vi "DPS_Statemachine.vi"() -> ()   [LabVIEW 2015]
uses:
  <vilib>/express/express arith-compare/Formula/XNode/ExpressFormulaBlockNode.xnode
  State_DPS.ctl
  <vilib>/myRIO/Express VI/Onboard IO/I2C/I2C Express VI.xnode
  <vilib>/myRIO/Instrument Drivers/Onboard IO/I2C/vis/Configure.vi
  <vilib>/myRIO/Instrument Drivers/Onboard IO/I2C/I2C.lvlib
  <vilib>/myRIO/Instrument Drivers/Onboard IO/I2C/vis/Write.vi
  <vilib>/myRIO/Instrument Drivers/Onboard IO/I2C/typedefs/I2C Transfer Rate.ctl
  <vilib>/myRIO/Instrument Drivers/Onboard IO/I2C/typedefs/I2C User Configuration.ctl
  <vilib>/myRIO/Instrument Drivers/Onboard IO/I2C/typedefs/I2C Configuration.ctl
  <vilib>/myRIO/Common/Instrument Driver Framework/myRIO v1.0/I2C/typedefs/I2C Channels Enum.ctl
  <vilib>/myRIO/Common/Instrument Driver Framework/Utilities/typedefs/Generic FPGA Reference.ctl
  <vilib>/myRIO/Common/Instrument Driver Framework/Utilities/typedefs/myRIO v1.0 Reference.ctl
  <vilib>/myRIO/Common/Instrument Driver Framework/Utilities/typedefs/Hardware Version Enum.ctl
  <vilib>/myRIO/Common/Instrument Driver Framework/Utilities/typedefs/myRIO Generic Hardware Reference.ctl
  <vilib>/myRIO/Instrument Drivers/Onboard IO/I2C/typedefs/I2C Reference.ctl
  <vilib>/myRIO/Instrument Drivers/Onboard IO/I2C/vis/myRIO I2C Open.xnode
  <vilib>/myRIO/Common/Instrument Driver Framework/Utilities/vis/Is FPGA Ref Available.vi
  <vilib>/myRIO/Common/Instrument Driver Framework/myRIO v1.0/I2C/vis/myRIO v1.1 Open I2C.vi
  <vilib>/userdefined/High Color/nirio_resource_hc.ctl
panel:
  out "I2C error":errorcluster
  out "True Pressure":dbl
  in  "stop":bool
  out "True Temperature":dbl
  out "Uncompensated P":dbl
  in  "XLSB Read":dbl
  in  "OSS":dbl
  in  "MSB Read":dbl format="%#_13g"
  in  "LSB Read":dbl
  out "Uncompensated T":dbl format="%#_13g"
  out "error out":errorcluster
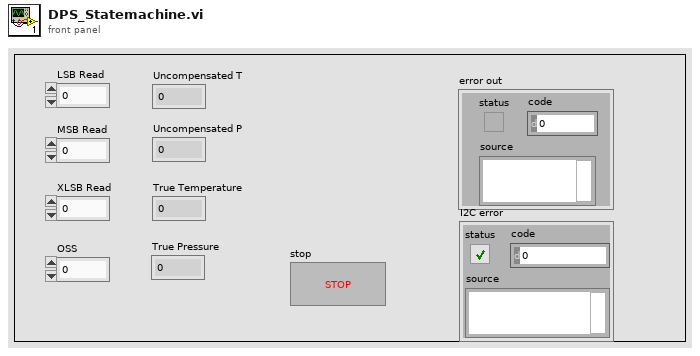
[diagram p1: front panel]
types:
  T1 = typedef "State_DPS.ctl" = enum16{"Read UT", "Wait", "Read & Calc UT", "Read UP", "Read & Calc UP", "Calculate TT", "Calculate TP"}
  T2 = typedef "I2C.lvlib/I2C Reference.ctl" = cluster{"myRIO Reference":T3, "I2C Channels Enum":T7, "I2C Configuration":T8}
  T3 = typedef "myRIO Generic Hardware Reference.ctl" = cluster{"myRIO Model":T4, "myRIO Hardware Reference":T5}
  T4 = typedef "Hardware Version Enum.ctl" = enum16{"Unknown", "myRIO-1900", "myRIO-1950", "roboRIO"}
  T5 = typedef "myRIO v1.0 Reference.ctl" = cluster{"Generic FPGA Reference":T6, "Allow multiple opens":bool}
  T6 = typedef "Generic FPGA Reference.ctl" = refnum<k20>
  T7 = typedef "I2C Channels Enum.ctl" = enum16{"Not Connected", "A/I2C", "B/I2C", "I2C/I2C"}
  T8 = typedef "I2C.lvlib/I2C Configuration.ctl" = cluster{"I2C Transfer Rate":T9}
  T9 = typedef "I2C.lvlib/I2C Transfer Rate.ctl" = enum16{"Standard mode (100 kbps)", "Fast mode (400 kbps)"}
  T10 = typedef "I2C.lvlib/I2C User Configuration.ctl" = cluster{"I2C Transfer Rate":T9}
  T11 = typedef "nirio_resource_hc.ctl" = tag
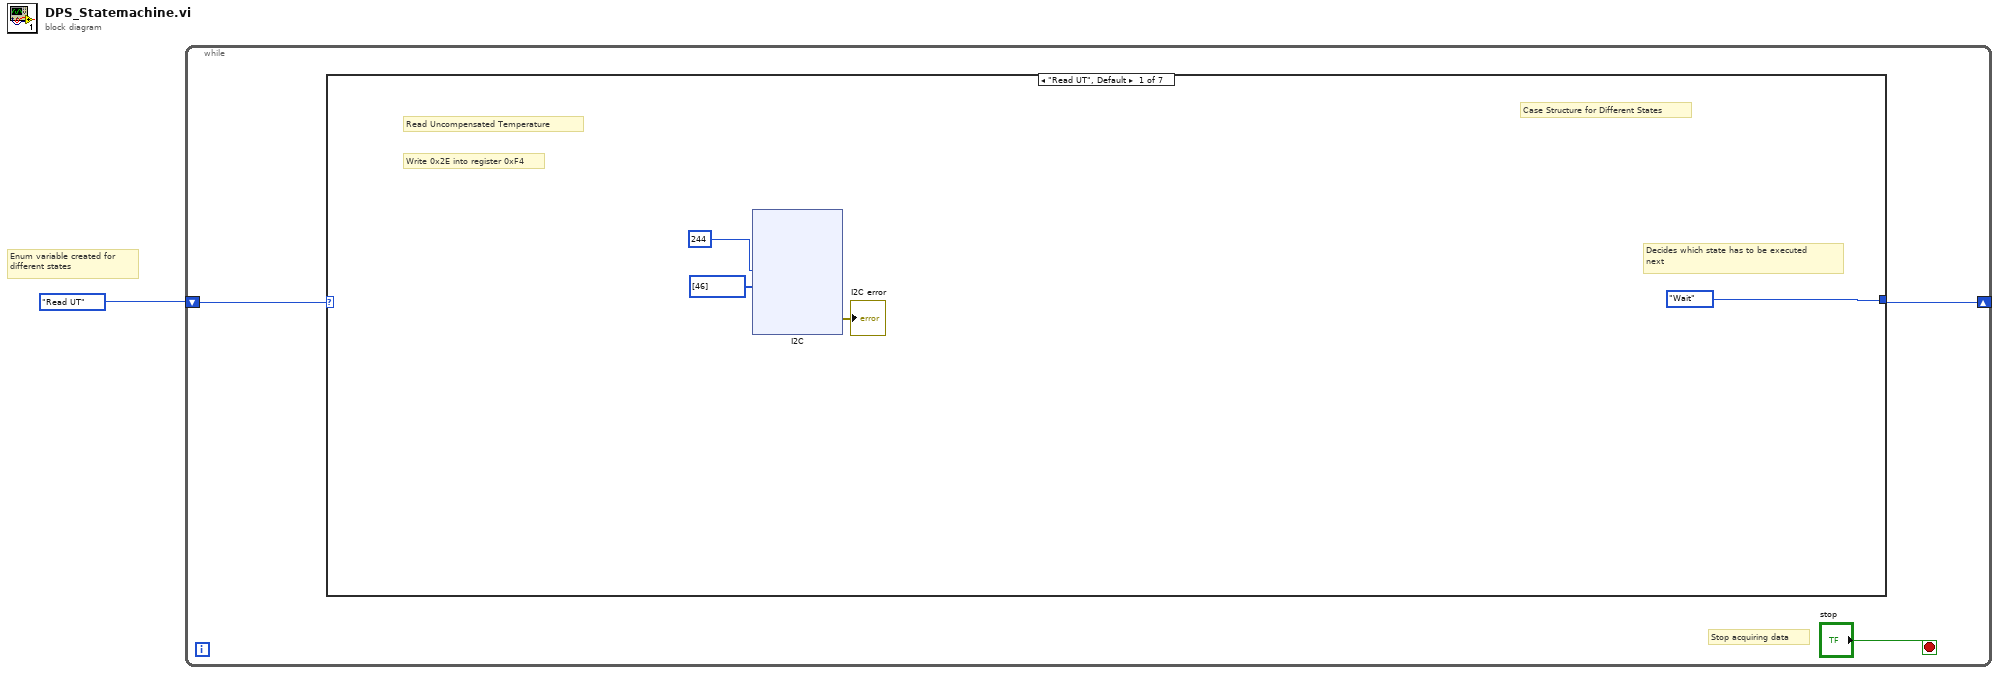
[diagram p0: block diagram]
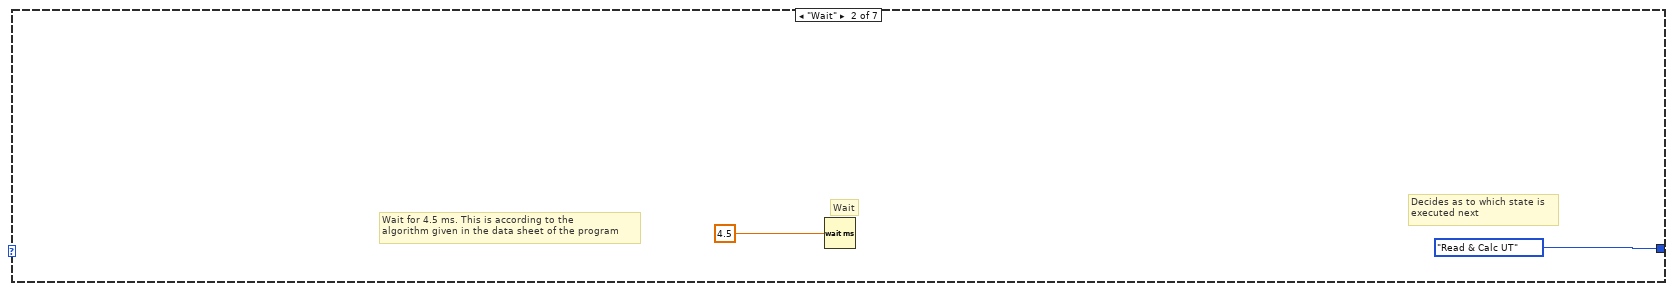
[diagram p2: hidden frame]
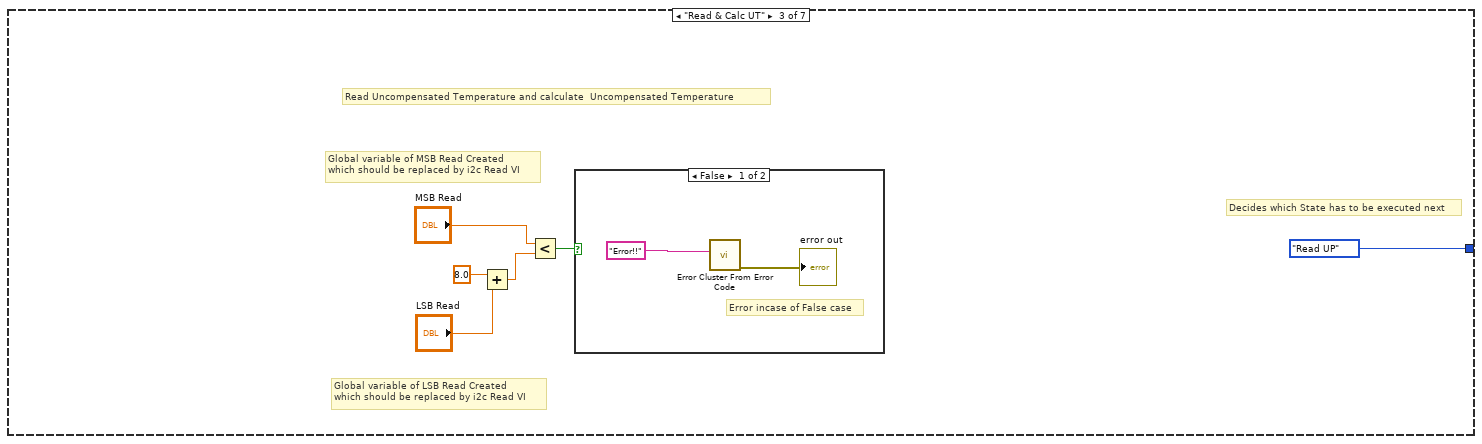
[diagram p3: hidden frame]
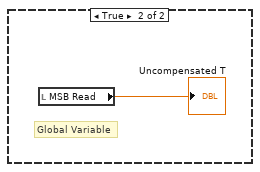
[diagram p4: hidden frame]
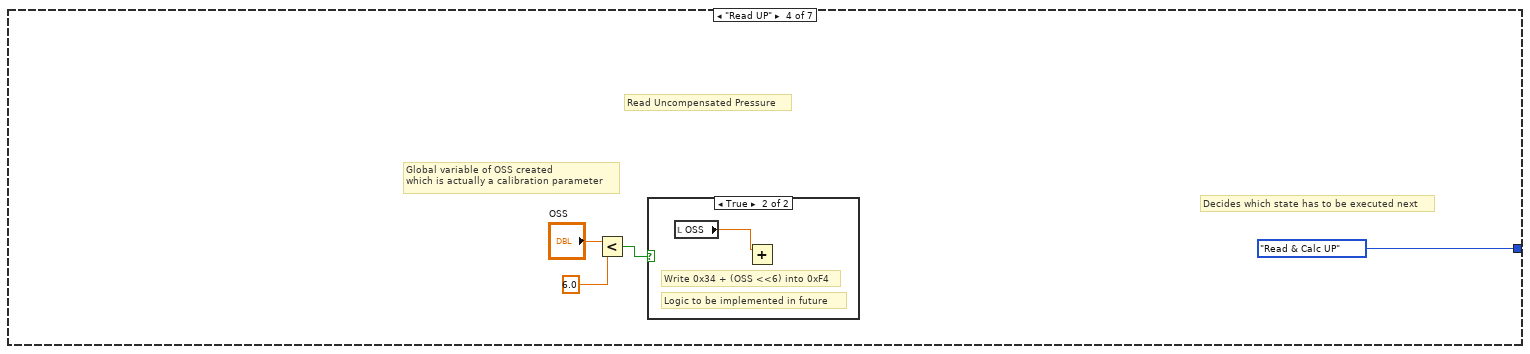
[diagram p5: hidden frame]
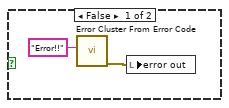
[diagram p6: hidden frame]
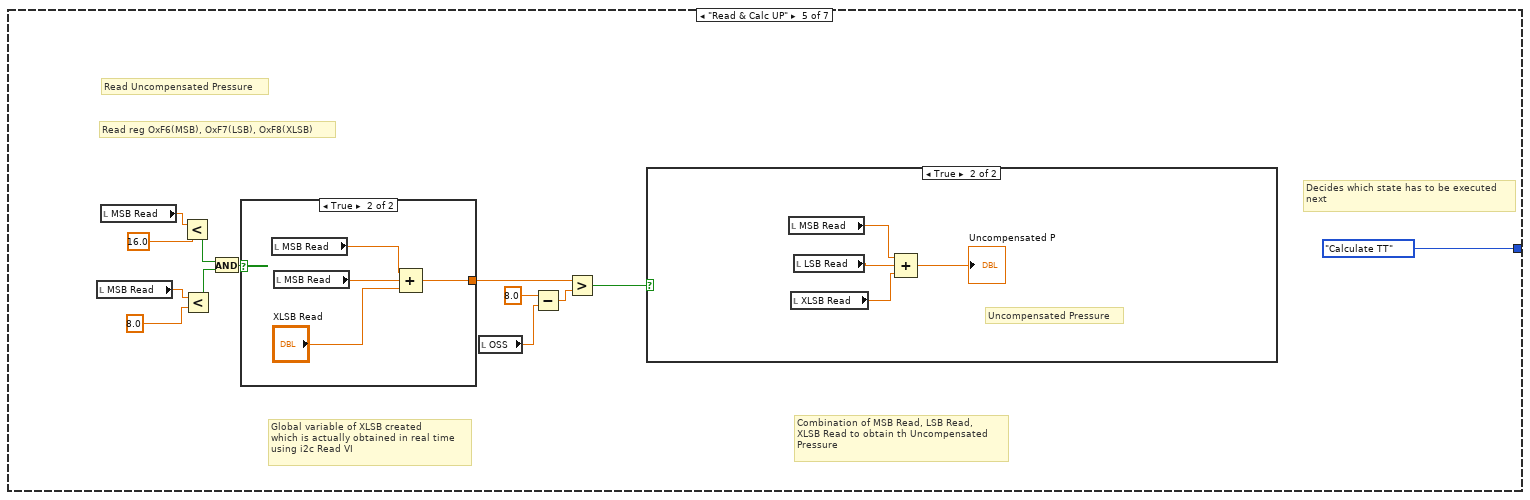
[diagram p7: hidden frame]
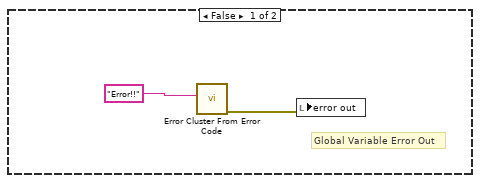
[diagram p8: hidden frame]
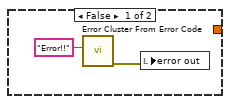
[diagram p9: hidden frame]
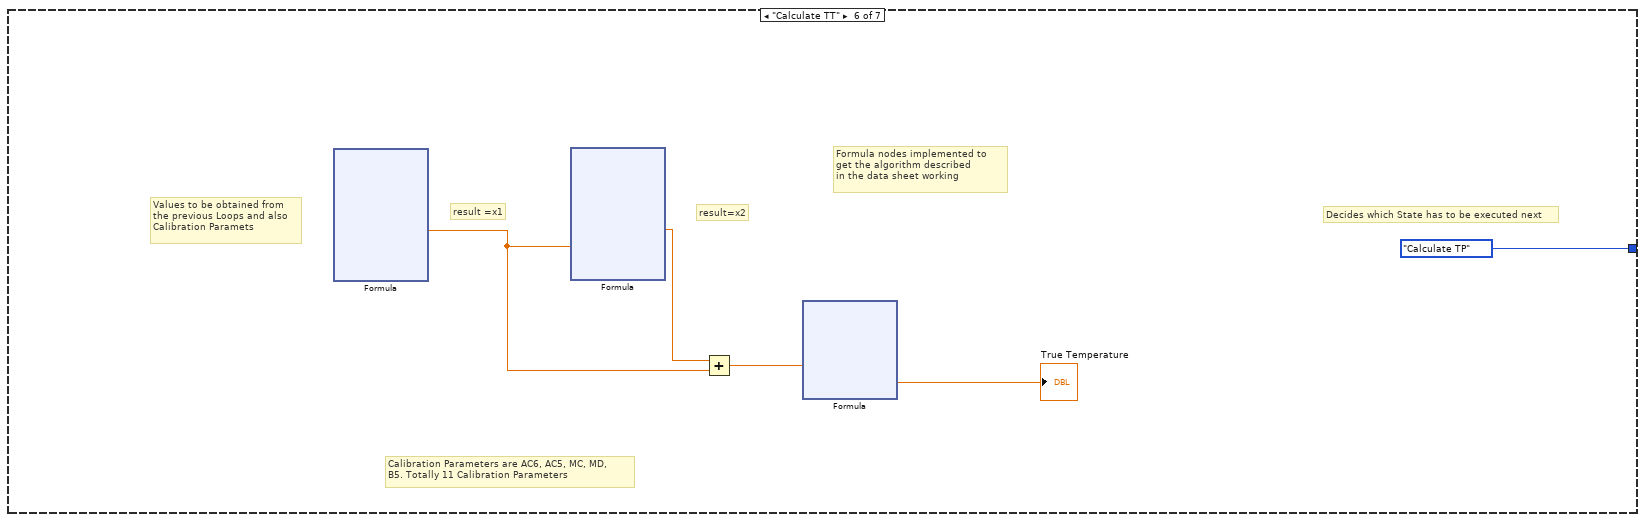
[diagram p10: hidden frame]
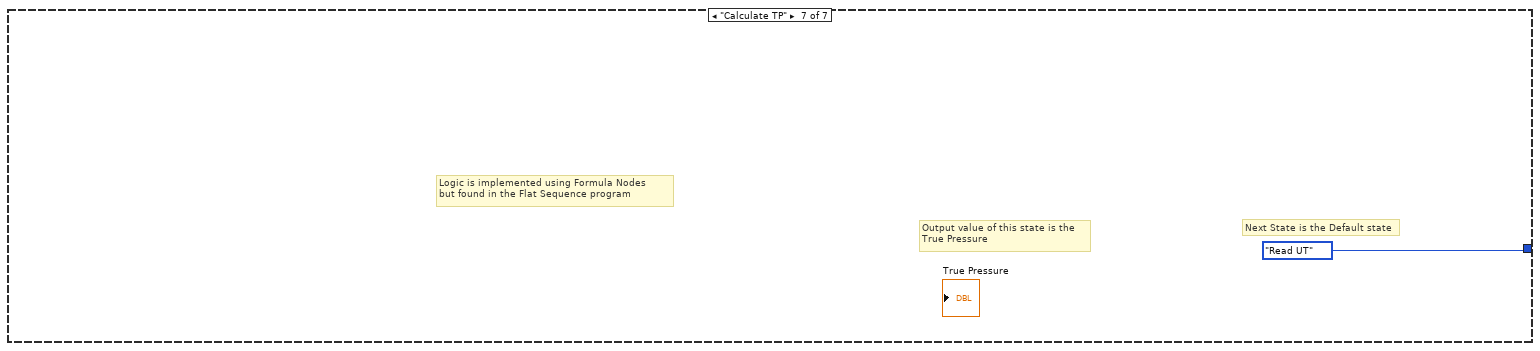
[diagram p11: hidden frame]
diagram:
  # "Enum variable created for\ndifferent states"
  n1 = while {
    shift-right: [w2] -> _
    shift-left: State_DPS."Read UT" ("State") -> [w3]
    stop <- "stop" stop-if-true
    # "Stop acquiring data"
    n2 = case shown="\"Read UT\", Default" w3 {
      tunnel: [State_DPS."Wait" ("State") State_DPS."Read & Calc UT" ("State") State_DPS."Read UP" ("State") State_DPS."Read & Calc UP" ("State") State_DPS."Calculate TT" ("State") State_DPS."Calculate TP" ("State") State_DPS."Read UT" ("State")] -> w2
      frame "Read UT", Default {
        # "Case Structure for Different States"
        # "Decides which state has to be executed \nnext"
        # "Write 0x2E into register 0xF4"
        # "Read Uncompensated Temperature"
        n3 = xnode "I2C"("Slave Address (7-bit)"=u8 244, "Bytes to Write"=u8[] [46]) -> ("error out"=→"I2C error":errorcluster)  [unwired: 1 in]
      }
      frame "Wait" {
        # "Decides as to which state is \nexecuted next"
        # "Wait for 4.5 ms. This is according to the \nalgorithm given in the data sheet of the program"
        # "Wait"
        n4 = Wait (ms)(milliseconds to wait=4.5) -> ()  [unwired: 1 out]
      }
      frame "Read & Calc UT" {
        # "Decides which State has to be executed next"
        # "Global variable of LSB Read Created \nwhich should be replaced by i2c Read VI"
        # "Global variable of MSB Read Created \nwhich should be replaced by i2c Read VI"
        # "Read Uncompensated Temperature and calculate  Uncompensated Temperature"
        n5 = Add(x=8.0, y="LSB Read") -> (x+y=w50:dbl)
        n6 = Less?(x="MSB Read", y=w50) -> (x < y?=w54:bool)
        n7 = case shown="False" w54 {
          frame False {
            # "Error incase of False case"
            n8 = call <vilib>:"Error Cluster From Error Code.vi"("error message (\"\")"="Error!!" ("error message (\"\")")) -> ("error out"=→"error out":errorcluster)  [unwired: 8 in]
          }
          frame True {
            # "Global Variable"
            n9 = local read "MSB Read"() -> (→"Uncompensated T":dbl)
          }
        }
      }
      frame "Read UP" {
        # "Decides which state has to be executed next"
        # "Global variable of OSS created \nwhich is actually a calibration parameter"
        # "Read Uncompensated Pressure"
        n10 = Less?(x="OSS", y=6.0) -> (x < y?=w59:bool)
        n11 = case shown="True" w59 {
          frame False {
            n12 = call <vilib>:"Error Cluster From Error Code.vi"("error message (\"\")"="Error!!" ("error message (\"\")")) -> ("error out"=w62:errorcluster)  [unwired: 8 in]
            n13 = local write "error out"(w62) -> ()
          }
          frame True {
            # "Logic to be implemented in future"
            # "Write 0x34 + (OSS <<6) into 0xF4"
            n14 = local read "OSS"() -> (w64:dbl)
            n15 = Add(x=w64) -> ()  [unwired: 1 in, 1 out]
          }
        }
      }
      frame "Read & Calc UP" {
        # "Combination of MSB Read, LSB Read,\nXLSB Read to obtain th Uncompensated\nPressure"
        # "Global variable of XLSB created \nwhich is actually obtained in real time\nusing i2c Read VI"
        # "Decides which state has to be executed \nnext"
        # "Read reg OxF6(MSB), OxF7(LSB), OxF8(XLSB)"
        # "Read Uncompensated Pressure"
        n16 = local read "MSB Read"() -> (w76:dbl)
        n17 = local read "MSB Read"() -> (w75:dbl)
        n18 = Less?(x=w75, y=16.0) -> (x < y?=w69:bool)
        n19 = Less?(x=w76, y=8.0) -> (x < y?=w70:bool)
        n20 = And(x=w69, y=w70) -> (x .and. y?=w68:bool)
        n21 = case shown="True" w68 {
          tunnel: [_ w88] -> w71
          frame False {
            n22 = call <vilib>:"Error Cluster From Error Code.vi"("error message (\"\")"="Error!!" ("error message (\"\")")) -> ("error out"=w84:errorcluster)  [unwired: 8 in]
            n23 = local write "error out"(w84) -> ()
          }
          frame True {
            n24 = local read "MSB Read"() -> (w87:dbl)
            n25 = local read "MSB Read"() -> (w86:dbl)
            n26 = Compound Arithmetic op=ADD(w87, w86, "XLSB Read") -> (w88:dbl)
          }
        }
        n27 = local read "OSS"() -> (w77:dbl)
        n28 = Subtract(x=8.0, y=w77) -> (x-y=w73:dbl)
        n29 = Greater?(x=w71, y=w73) -> (0:w74:bool)
        n30 = case shown="True" w74 {
          frame False {
            # "Global Variable Error Out"
            n31 = call <vilib>:"Error Cluster From Error Code.vi"("error message (\"\")"="Error!!" ("error message (\"\")")) -> ("error out"=w78:errorcluster)  [unwired: 8 in]
            n32 = local write "error out"(w78) -> ()
          }
          frame True {
            # "Uncompensated Pressure"
            n33 = local read "MSB Read"() -> (w81:dbl)
            n34 = local read "XLSB Read"() -> (w82:dbl)
            n35 = local read "LSB Read"() -> (w80:dbl)
            n36 = Compound Arithmetic op=ADD(w81, w80, w82) -> (→"Uncompensated P":dbl)
          }
        }
      }
      frame "Calculate TT" {
        # "Formula nodes implemented to \nget the algorithm described \nin the data sheet working"
        # "Decides which State has to be executed next"
        # "Calibration Parameters are AC6, AC5, MC, MD,\nB5. Totally 11 Calibration Parameters"
        # "Values to be obtained from \nthe previous Loops and also\nCalibration Paramets"
        # "result=x2"
        # "result =x1"
        n37 = xnode "Formula"() -> ("Result"=w93:dbl)  [unwired: 4 in, 1 out]
        n38 = xnode "Formula"("Result1"=w93) -> ("Result"=w94:dbl)  [unwired: 3 in, 1 out]
        n39 = Add(x=w94, y=w93) -> (x+y=w92:dbl)
        n40 = xnode "Formula"("B5"=w92) -> ("Result"=→"True Temperature":dbl)  [unwired: 1 in, 1 out]
      }
      frame "Calculate TP" {
        # "Next State is the Default state"
        # "Output value of this state is the \nTrue Pressure"
        # "Logic is implemented using Formula Nodes \nbut found in the Flat Sequence program"
      }
    }
  }
